vi "F_B_SWLDA_Calculator.vi"(0 "LDA_matrix":path caption="LDA_matrix.txt", 1 "Flash_Repeat":i32=20, 5 "Weight":path caption="weight.txt", 7 "Target_order.txt":path, 9 "mius_flash_order":path, 11 "Brain":path, 12 "피험자이름":string="홍길동") -> (4 "ERP_발생_total":i16[](array[numeric]), 15 "ACC(%)":dbl)   [LabVIEW 2014]
uses:
  <vilib>/Utility/file.llb/Read From Spreadsheet File (DBL).vi
  <vilib>/Analysis/Matrix/Numeric/Conversions/Array To Matrix - RA2.vi
  <vilib>/Analysis/Matrix/Numeric/Conversions/Array To Matrix - RA.vi
  <vilib>/Utility/file.llb/Read From Spreadsheet File (I64).vi
  <vilib>/Utility/file.llb/Write To Spreadsheet File (I64).vi
  <vilib>/Utility/file.llb/Write To Spreadsheet File (DBL).vi
  <vilib>/Utility/file.llb/Write To Spreadsheet File (string).vi
  <vilib>/Analysis/Matrix/NI_Matrix.lvlib
panel:
  out "ACC":i16
  in  "Channel selection":bool[](array[boolean])=[TRUE, TRUE, TRUE, TRUE, TRUE, TRUE, TRUE, TRUE, TRUE, TRUE, TRUE]
  out "Target_order":i64[](array[numeric])
  out "Selected_Target":i32[](array[numeric])
  out "Accuracy":i16[](array[numeric])
  in  "사용할 Parameter 갯수":i32=4
  out "error out":errorcluster
  in  "Random_num":i32=9
  in  "Frame_Length":i32=25
  in  "Sampling_Rate":dbl=500.0
  in  "ERP_Parameters_of_NonTarget":path caption="ERP_Parameters_of_NonTarget.txt"
  in  "ERP_Parameters_of_Target":path caption="ERP_Parameters_of_Target.txt"
  # "ERP_Parameter안씀. LDA바로 집어넣으면 됨"
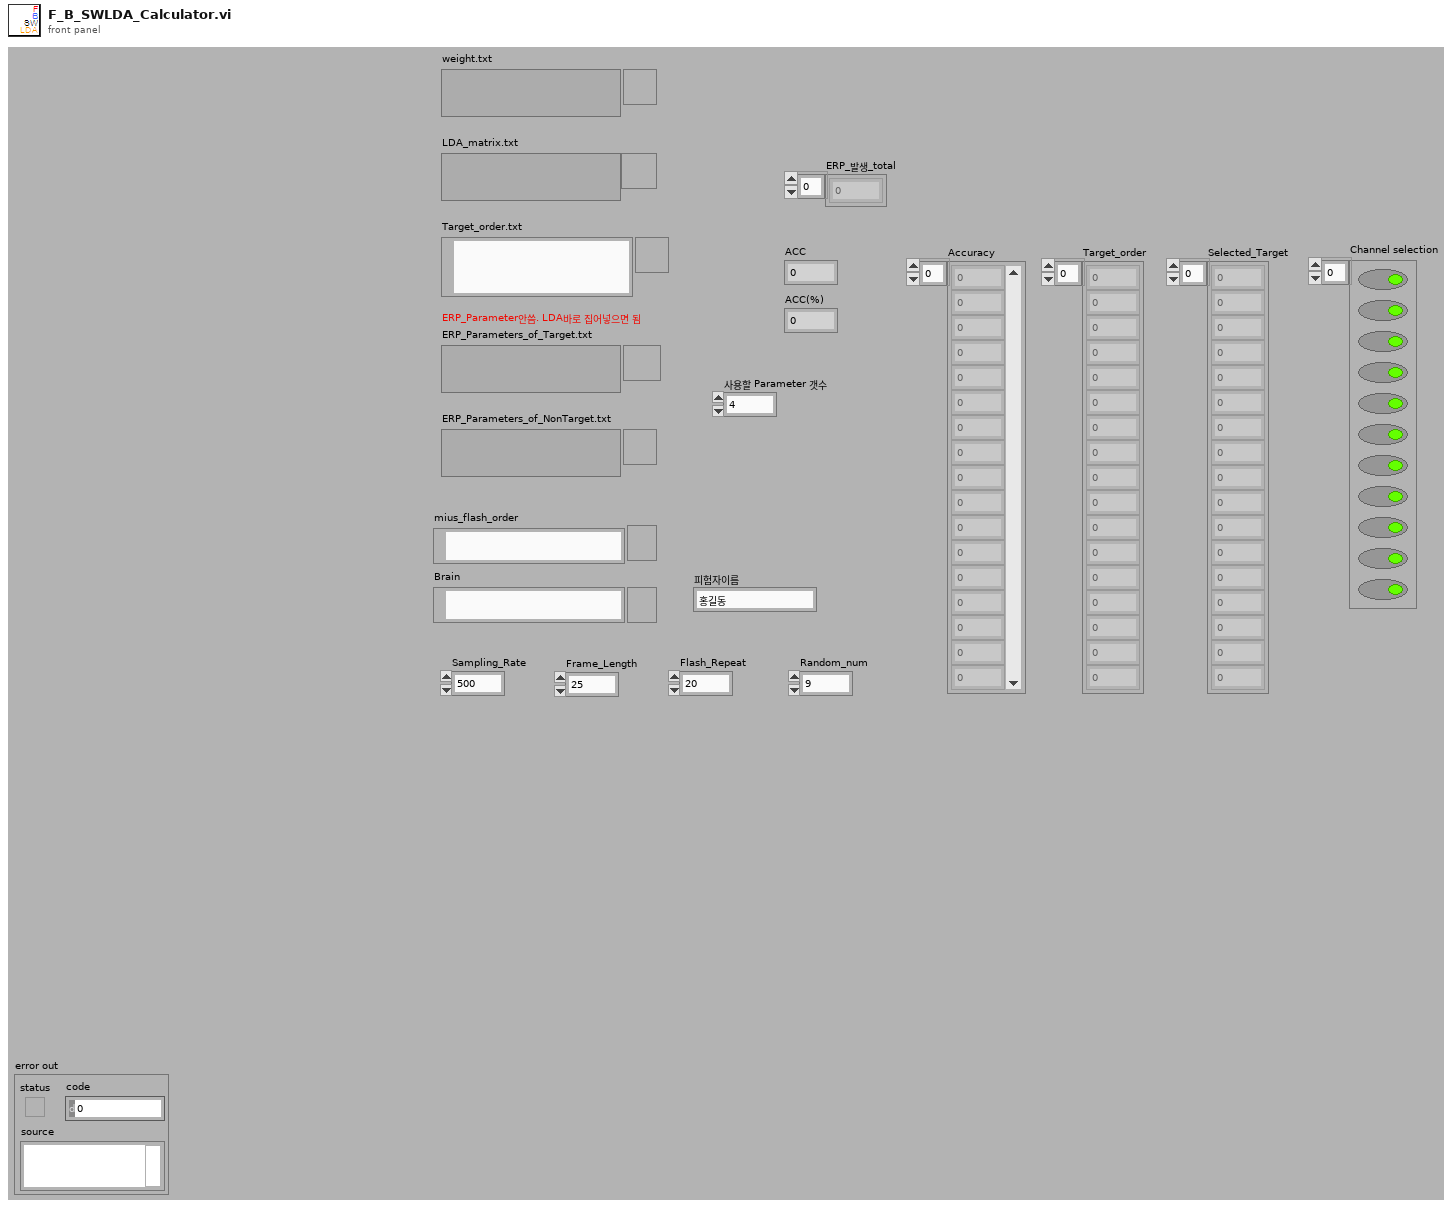
[diagram p1: front panel]
types:
  T1 = typedef "NI_Matrix.lvlib/RealMatrix.ctl" = dbl[][]
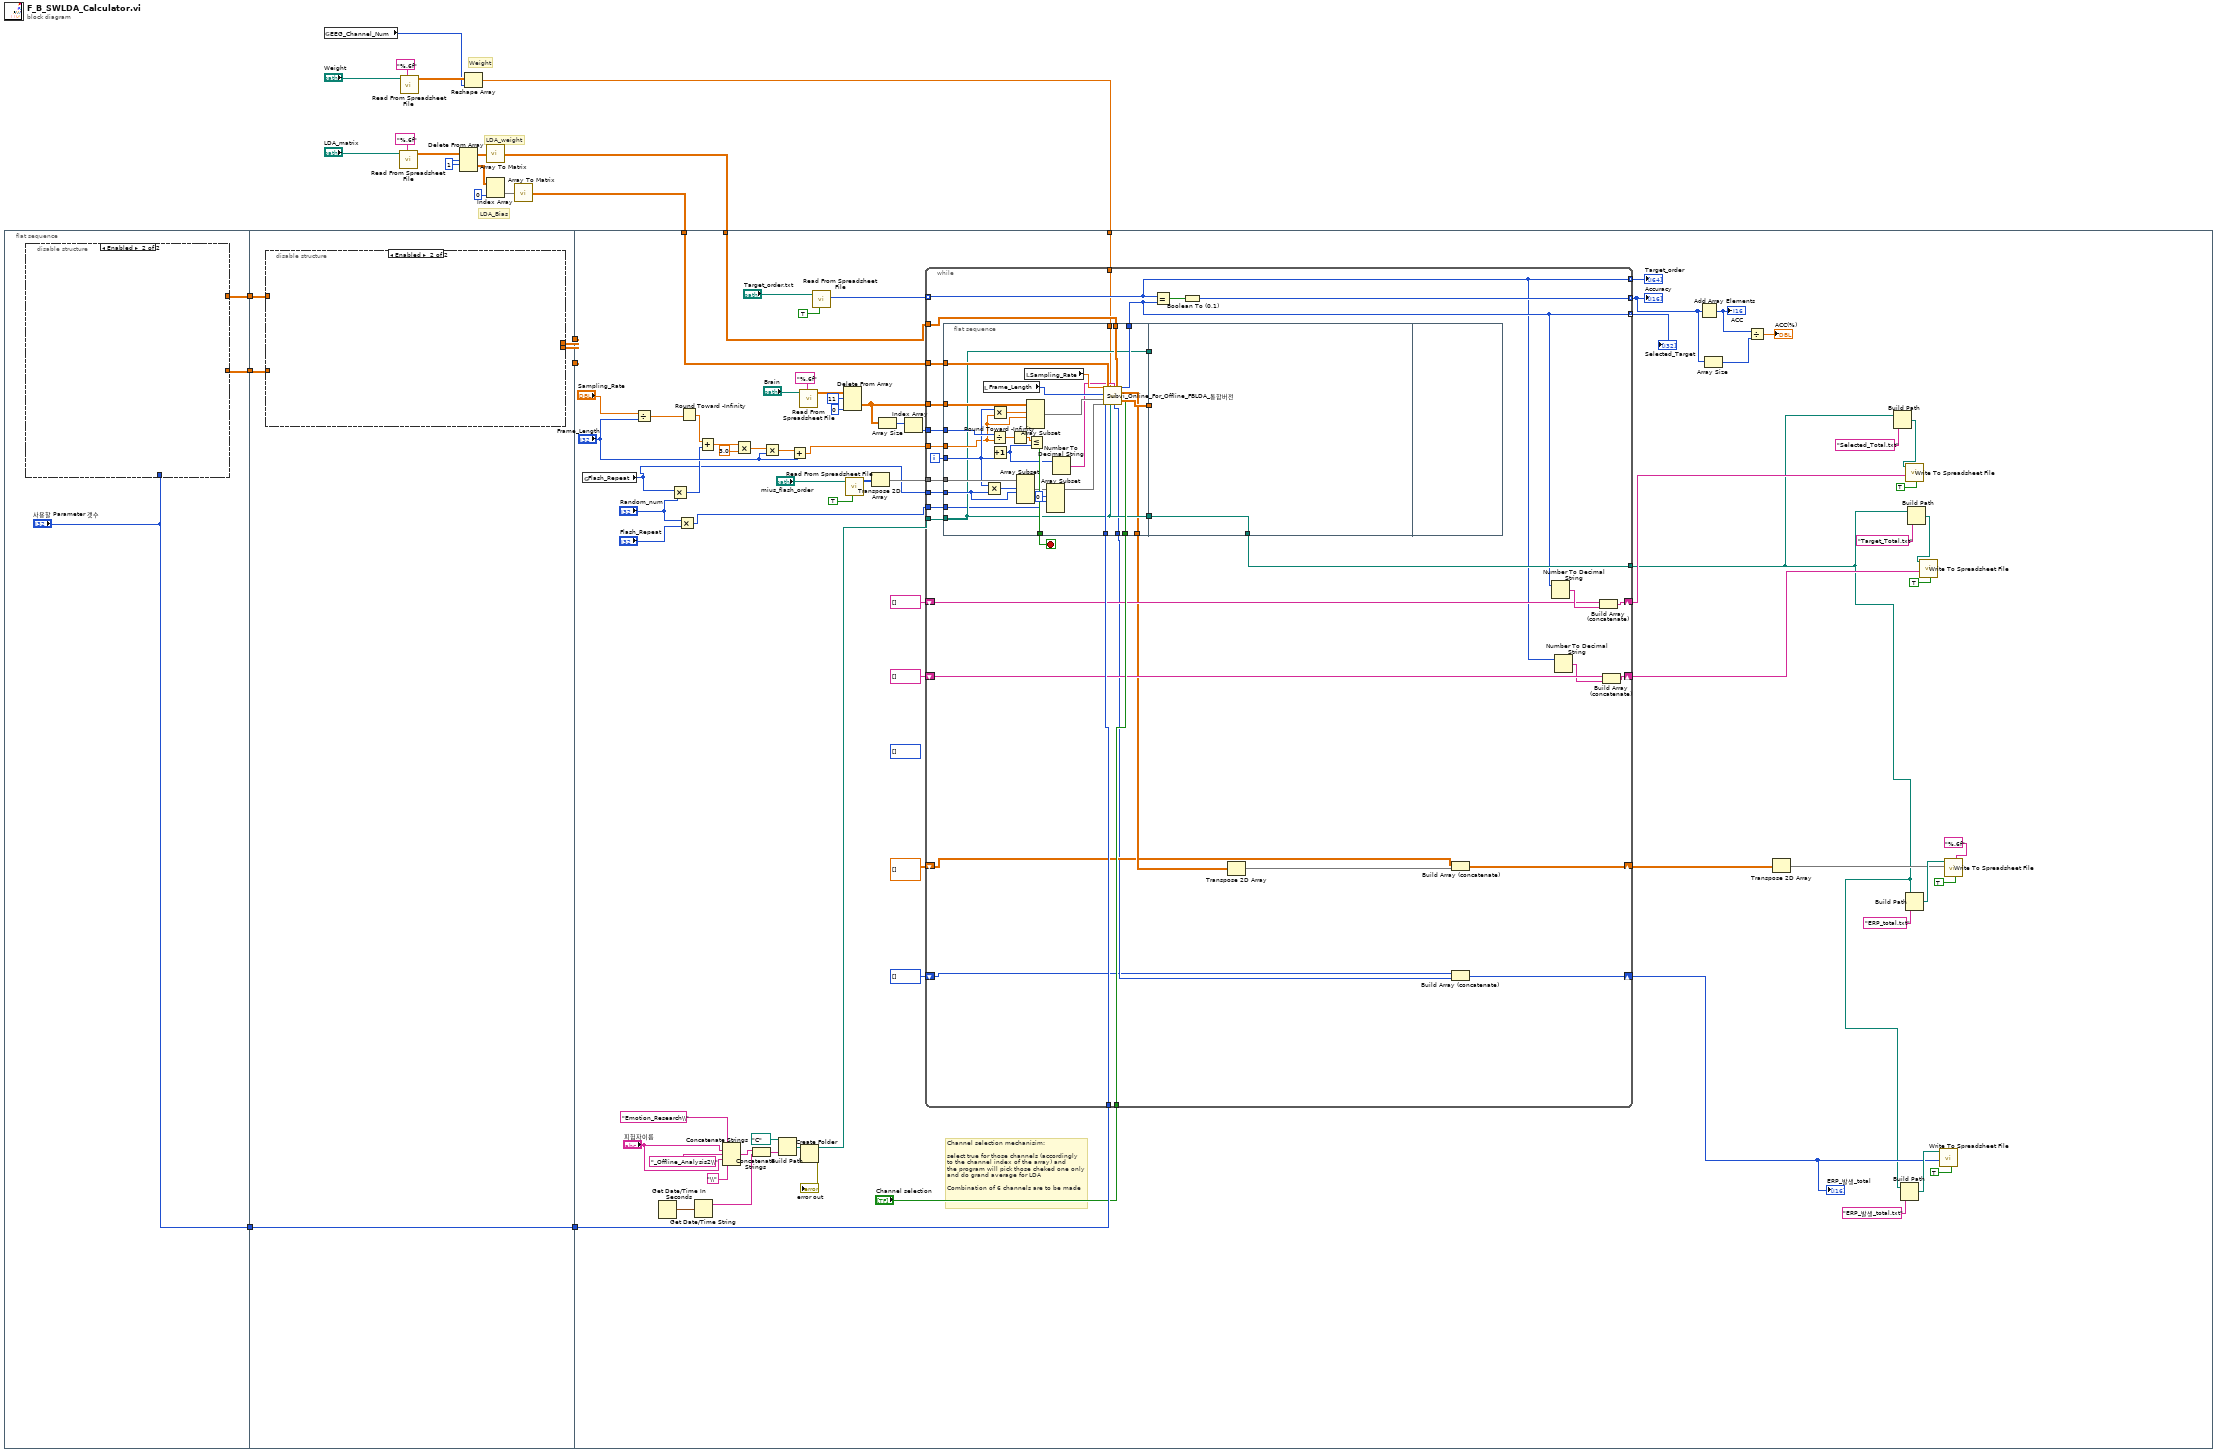
[diagram p0: block diagram]
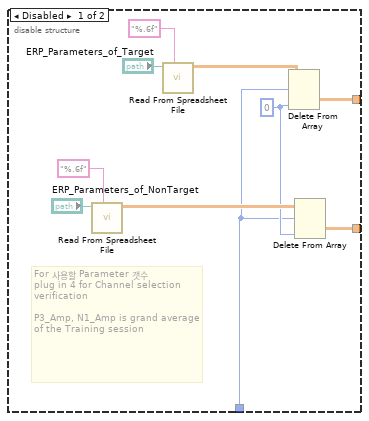
[diagram p2: hidden frame]
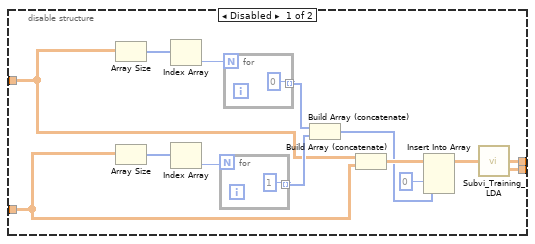
[diagram p3: hidden frame]
diagram:
  w10 = 1 ("인덱스 (행)")
  # "LDA_Bias"
  # "LDA_weight"
  # "Weight"
  n1 = flat-sequence {
    tunnel: [w24] -> w21
    tunnel: [w23] -> w20
    tunnel: ["사용할 Parameter 갯수"] -> w17
    tunnel: w21 -> [w39]
    tunnel: w20 -> [w38]
    tunnel: [w37] -> w19
    tunnel: [w36] -> w18
    tunnel: w17 -> [w35]
    tunnel: [w35] -> w16
    tunnel: w19 -> [_]
    tunnel: w18 -> [_]
    tunnel: w16 -> [w99]
    tunnel: w7 -> [w70]
    tunnel: w6 -> [w69]
    tunnel: w1 -> [w68]
    frame #0 {
      n2 = disable-structure shown="Enabled" {
        disable-tunnel: [w27 _] -> w24
        disable-tunnel: [w26 _] -> w23
        disable-tunnel: "사용할 Parameter 갯수" -> [w25 _]
        frame Disabled {
          w28 = 0 ("비활성화된 인덱스 (열)")
          # "For 사용할 Parameter 갯수\nplug in 4 for Channel selection\nverification\n\nP3_Amp, N1_Amp is grand average of the Training session"
          n3 = call-poly <vilib>:"Read From Spreadsheet File.vi"("format (%.3f)"="%.6f", "file path (dialog if empty)"="ERP_Parameters_of_NonTarget") -> ("all rows"=w29:dbl[][])  [unwired: 5 in, 4 out]
          n4 = call-poly <vilib>:"Read From Spreadsheet File.vi"("format (%.3f)"="%.6f", "file path (dialog if empty)"="ERP_Parameters_of_Target") -> ("all rows"=w30:dbl[][])  [unwired: 5 in, 4 out]
          n5 = Delete From Array(array=w30, length=w25, index (col)=w28) -> (deleted portion=w27:dbl[][])  [unwired: 1 in, 1 out]
          n6 = Delete From Array(array=w29, length=w25, index (col)=w28) -> (deleted portion=w26:dbl[][])  [unwired: 1 in, 1 out]
        }
        frame Enabled {
        }
      }
    }
    frame #1 {
      n7 = disable-structure shown="Enabled" {
        disable-tunnel: w39 -> [w44 _]
        disable-tunnel: w38 -> [w43 _]
        disable-tunnel: [w42 _] -> w37
        disable-tunnel: [w41 _] -> w36
        frame Disabled {
          n8 = Array Size(array=w44) -> (size(s)=w48:i32[])
          n9 = Array Size(array=w43) -> (size(s)=w49:i32[])
          n10 = Index Array(array=w48) -> (element=w50:i32)  [unwired: 1 in]
          n11 = Index Array(array=w49) -> (element=w51:i32)  [unwired: 1 in]
          n12 = for {
            N: w51 -> [_]
            tunnel: [1] -> w53 mode=indexing
          }
          n13 = for {
            N: w50 -> [_]
            tunnel: [0] -> w52 mode=indexing
          }
          n14 = Build Array (concatenate)(w52, w53) -> (w45:i32[])
          n15 = Build Array (concatenate)(w44, w43) -> (w46:dbl[][])
          n16 = Insert Into Array(array=w46, index (col)=0 ("비활성화된 인덱스 (열)"), new element=w45) -> (w40:dbl[][])  [unwired: 1 in]
          n17 = call "Subvi_Training_LDA.vi"("Input_Data"=w40) -> ("A * B 2"=w42:T1, "A * B"=w41:T1)
        }
        frame Enabled {
        }
      }
    }
    frame #2 {
      (unwired) i16[] []
      # "Channel selection mechanisim:\n\nselect true for those channels (accordingly\nto the channel index of the array) and \nthe program will pick those cheked one only\nand do grand average for LDA\n\nCombination of 6 channels are to be made"
      n18 = global read "Control_Panel.vi" "Flash_Repeat"() -> (w59:i32)
      n19 = Divide(x="Sampling_Rate", y="Frame_Length") -> (x/y=w111:dbl)
      n20 = Get Date/Time In Seconds() -> (seconds since 1Jan1904=w122:timestamp)
      n21 = Multiply(x=w59, y="Random_num") -> (x*y=w113:i32)
      n22 = Multiply(x="Random_num", y="Flash_Repeat") -> (x*y=w56:i32)
      n23 = Round Toward -Infinity(1:w111) -> (0:w112:dbl)
      n24 = Get Date/Time String(seconds (now)=w122) -> (date string=w121:string)  [unwired: 2 in, 1 out]
      n25 = Add(x=w112, y=w113) -> (x+y=w114:dbl)
      n26 = Concatenate Strings("Emotion_Research\\" ("string"), "피험자이름", "_Offline_Analysis2\\" ("문자열"), "피험자이름", "\\" ("string")) -> (w126:string)
      n27 = Multiply(x=w114, y=3.0) -> (x*y=w116:dbl)
      n28 = Concatenate Strings(w126, w121) -> (w124:string)
      n29 = Multiply(x=w116, y="Frame_Length") -> (x*y=w118:dbl)
      n30 = Build Path(base path=path "C:/" ("path"), name or relative path=w124) -> (appended path=w123:path)
      n31 = Add(x=w118, y="Frame_Length") -> (x+y=w119:dbl)
      n32 = call-poly <vilib>:"Read From Spreadsheet File.vi"("format (%.3f)"="%.6f", "file path (dialog if empty)"="Brain") -> ("all rows"=w104:dbl[][])  [unwired: 5 in, 4 out]
      n33 = Create Folder(path (use dialog)=w123) -> (created path=w128:path, error out=→"error out":errorcluster)  [unwired: 2 in, 1 out]
      n34 = call-poly <vilib>:"Read From Spreadsheet File.vi"("transpose (no:F)"=TRUE, "file path (dialog if empty)"="Target_order.txt") -> ("first row"=w97:i64[])  [unwired: 5 in, 4 out]
      n35 = Delete From Array(array=w104, length=11 ("길이"), index (col)=0 ("비활성화된 인덱스 (열)")) -> (deleted portion=w107:dbl[][])  [unwired: 1 in, 1 out]
      n36 = call-poly <vilib>:"Read From Spreadsheet File.vi"("transpose (no:F)"=TRUE, "file path (dialog if empty)"="mius_flash_order") -> ("all rows"=w106:i64[][])  [unwired: 5 in, 4 out]
      n37 = Transpose 2D Array(2D array=w106) -> (transposed array=w60:i64[][])
      n38 = Array Size(array=w107) -> (size(s)=w108:i32[])
      n39 = Index Array(array=w108) -> (element=w109:i32)  [unwired: 1 in]
      n40 = while {
        tunnel: w69 -> [w165]
        tunnel: w70 -> [w164]
        tunnel: w107 -> [w162]
        tunnel: w60 -> [w161]
        tunnel: w109 -> [w163]
        tunnel: w119 -> [w159]
        tunnel: w59 -> [w160]
        tunnel: w128 -> [w156]
        tunnel: w99 -> [w154]
        tunnel: w97 -> [w143] mode=indexing
        tunnel: [w152] -> w64 mode=indexing
        tunnel: [w143] -> w94 mode=indexing
        tunnel: [w144] -> w95 mode=indexing
        tunnel: "Channel selection" -> [w149]
        tunnel: [w148] -> w67
        shift-right: [w146] -> w84
        shift-left: string[] [] -> [w145]
        shift-right: [w142] -> w83
        shift-left: string[] [] -> [w141]
        shift-right: [w138] -> w78
        shift-left: dbl[][] [] -> [w137]
        shift-right: [w135] -> w71
        shift-left: i16[] [] -> [w134]
        tunnel: w68 -> [w133]
        tunnel: w56 -> [w131]
        i -> [w151]
        stop <- w150 stop-if-true
        n41 = flat-sequence {
          tunnel: w165 -> [w195]
          tunnel: w164 -> [w194]
          tunnel: w163 -> [w193]
          tunnel: [w192] -> w150
          tunnel: w162 -> [w191]
          tunnel: w161 -> [w188]
          tunnel: w160 -> [w186]
          tunnel: w151 -> [w184]
          tunnel: w159 -> [w183]
          tunnel: [w177] -> w158
          tunnel: w156 -> [w173]
          tunnel: [w173] -> w157
          tunnel: [w173] -> w155
          tunnel: w154 -> [w176]
          tunnel: [w175] -> w144
          tunnel: w149 -> [w174]
          tunnel: [w172] -> w140
          tunnel: [w170] -> w136
          tunnel: w133 -> [w169]
          tunnel: w131 -> [w166]
          tunnel: w158 -> [_]
          tunnel: w157 -> [_]
          tunnel: w155 -> [w196]
          tunnel: [w196] -> w148
          frame #0 {
            n42 = local read "Frame_Length"() -> (w179:i32)
            n43 = Multiply(x=w184, y=w186) -> (x*y=w187:i32)
            n44 = Divide(x=w193, y=w183) -> (x/y=w182:dbl)
            n45 = Multiply(x=w184, y=w183) -> (x*y=w190:dbl)
            n46 = Increment(x=w184) -> (x+1=w178:i32)
            n47 = Round Toward -Infinity(1:w182) -> (0:w181:dbl)
            n48 = Array Subset(array=w188, index (row)=w187, length (row)=w186) -> (w185:i64[][])  [unwired: 2 in]
            n49 = local read "Sampling_Rate"() -> (w180:dbl)
            n50 = Array Subset(array=w191, index (row)=w190, length (row)=w183) -> (w189:dbl[][])  [unwired: 2 in]
            n51 = Less Or Equal?(x=w181, y=w178) -> (x <= y?=w192:bool)
            n52 = Array Subset(array=w185, index (row)=0 ("index"), length (row)=w166) -> (w168:i64[][])  [unwired: 2 in]
            n53 = Number To Decimal String(number=w178) -> (decimal integer string=w171:string)  [unwired: 1 in]
            n54 = call "Subvi_Online_For_Offline_FBLDA_통합버전.vi"("rate"=w180, "samples per channel"=w179, "Brain_data_source"=w189, "Target_Flash_Order"=w168, "Value"=w195, "사용할 Parameter 갯수"=w176, "Weight"=w169, "Path"=w173, "Number"=w171, "Matrix"=w194, "Channel selection"=w174) -> ("LDA_Parameter"=w177:dbl[][], "EPR_발생_total"=w170:i16[], "output-0~8"=w175:i32, "ERP_Parameters"=w172:dbl[][])  [unwired: 13 in]
          }
          frame #1 {
          }
          frame #2 {
          }
        }
        n55 = Equal?(x=w143, y=w144) -> (x = y?=w153:bool)
        n56 = Boolean To (0,1)(Boolean=w153) -> (0, 1=w152:i16)
        n57 = Transpose 2D Array(2D array=w140) -> (transposed array=w139:dbl[][])
        n58 = Build Array (concatenate)(w134, w136) -> (w135:i16[])
        n59 = Build Array (concatenate)(w137, w139) -> (w138:dbl[][])
        n60 = Number To Decimal String(number=w144) -> (decimal integer string=w147:string)  [unwired: 1 in]
        n61 = Number To Decimal String(number=w143) -> (decimal integer string=w132:string)  [unwired: 1 in]
        n62 = Build Array (concatenate)(w145, w147) -> (w146:string[])
        n63 = Build Array (concatenate)(w141, w132) -> (w142:string[])
      }
      "Accuracy" <- w64
      "Selected_Target" <- w95
      "Target_order" <- w94
      "ERP_발생_total" <- w71
      n64 = Add Array Elements(numeric array=w64) -> (sum=w63:i16)
      "ACC" <- w63
      n65 = Array Size(array=w64) -> (size(s)=w62:i32)
      n66 = Divide(x=w63, y=w62) -> (x/y=→"ACC(%)":dbl)
      n67 = Transpose 2D Array(2D array=w78) -> (transposed array=w76:dbl[][])
      n68 = Build Path(base path=w67, name or relative path="Selected_Total.txt") -> (appended path=w86:path)
      n69 = Build Path(base path=w67, name or relative path="ERP_발생_total.txt") -> (appended path=w73:path)
      n70 = call-poly <vilib>:"Write To Spreadsheet File.vi"("transpose? (no:F)"=TRUE, "1D data"=w84, "file path (dialog if empty)"=w86) -> ()  [unwired: 5 in, 1 out]
      n71 = Build Path(base path=w67, name or relative path="ERP_total.txt") -> (appended path=w79:path)
      n72 = Build Path(base path=w67, name or relative path="Target_Total.txt") -> (appended path=w91:path)
      n73 = call-poly <vilib>:"Write To Spreadsheet File.vi"("transpose? (no:F)"=TRUE, "1D data"=w83, "file path (dialog if empty)"=w91) -> ()  [unwired: 5 in, 1 out]
      n74 = call-poly <vilib>:"Write To Spreadsheet File.vi"("transpose? (no:F)"=TRUE, "1D data"=w71, "file path (dialog if empty)"=w73) -> ()  [unwired: 5 in, 1 out]
      n75 = call-poly <vilib>:"Write To Spreadsheet File.vi"("transpose? (no:F)"=TRUE, "format (%.3f)"="%.6f", "2D data"=w76, "file path (dialog if empty)"=w79) -> ()  [unwired: 4 in, 1 out]
    }
  }
  n76 = global read "Control_Panel.vi" "EEG_Channel_Num"() -> (w2:i32)
  n77 = call-poly <vilib>:"Read From Spreadsheet File.vi"("format (%.3f)"="%.6f", "file path (dialog if empty)"="LDA_matrix") -> ("all rows"=w8:dbl[][])  [unwired: 5 in, 4 out]
  n78 = call-poly <vilib>:"Read From Spreadsheet File.vi"("format (%.3f)"="%.6f", "file path (dialog if empty)"="Weight") -> ("all rows"=w3:dbl[][])  [unwired: 5 in, 4 out]
  n79 = Delete From Array(array=w8, length=w10, index (row)=w10) -> (deleted portion=w13:dbl[][], array with subset deleted=w12:dbl[][])  [unwired: 1 in]
  n80 = Reshape Array(w3, w2) -> (w1:dbl[])
  n81 = call-poly <vilib>:"Array To Matrix.vi"("Real 2D Array"=w12) -> ("Real Matrix"=w7:T1)
  n82 = Index Array(array=w13, index (col)=0 ("인덱스")) -> (element=w11:dbl[])  [unwired: 1 in]
  n83 = call-poly <vilib>:"Array To Matrix.vi"("Real 1D Array"=w11) -> ("Real Matrix (Column Vector)"=w6:T1)
